vi "SPI Slave Get Bytes.vi"(7 "BufferSize":i32, 9 "pReadData":u8[](array[numeric])=array[4097 elements], 10 "SPIIndex":i32, 11 "DevHandle":i32) -> (1 "pReadData out":u8[](array[numeric]), 3 "function return":i32)   [LabVIEW 2010, in "usb2spi.lvlib"]
doc: "int WINAPI SPI_SlaveGetBytes(int DevHandle,int SPIIndex,unsigned char *pReadData,int BufferSize);"
uses:
  usb2spi.lvlib
  USB2XXX/trunk/USB2XXX/USB2XXX/vs2010/Release/USB2XXX.dll
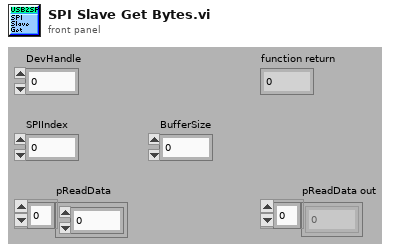
[diagram p1: front panel]
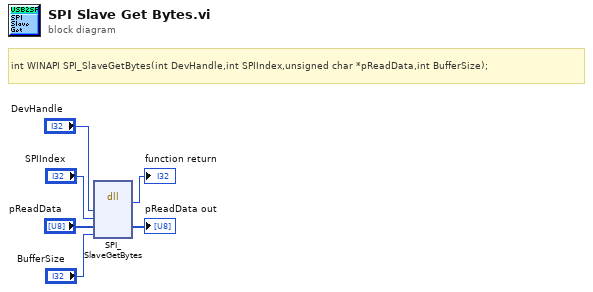
[diagram p0: block diagram]
diagram:
  # "int WINAPI SPI_SlaveGetBytes(int DevHandle,int SPIIndex,unsigned char *pReadData,int BufferSize);"
  n1 = dll-call lib="E:/OtherWork/STM32/USB2XXX/trunk/USB2XXX/USB2XXX/vs2010/Release/USB2XXX.*" fn="SPI_SlaveGetBytes"("DevHandle"="DevHandle", "SPIIndex"="SPIIndex", "pReadData"="pReadData", "BufferSize"="BufferSize") -> (→"function return":i32, "pReadData"=→"pReadData out":u8[])  [unwired: 6 in, 2 out]
